vi "NO_NO_HumanDriveButtonReefCoralPositions.vi"() -> ()   [LabVIEW 2023]
uses:
  <vilib>/Rock Robotics/WPI/ThirdParty/JAS_Junk/TrajLib/Trajectory_Library.lvlib
  HumanGlobal.vi
panel:
  in  "DriverBoxRight":bool
  in  "DriverBoxLeft":bool
  in  "19-6 (bottom left)":bool
  in  "20-11 (top left)":bool
  in  "21-10 (outer)":bool
  in  "22-9 (top right)":bool
  in  "17-8 (bottom right)":bool
  in  "18-7 (inner)":bool
  out "DriveTraj":bool
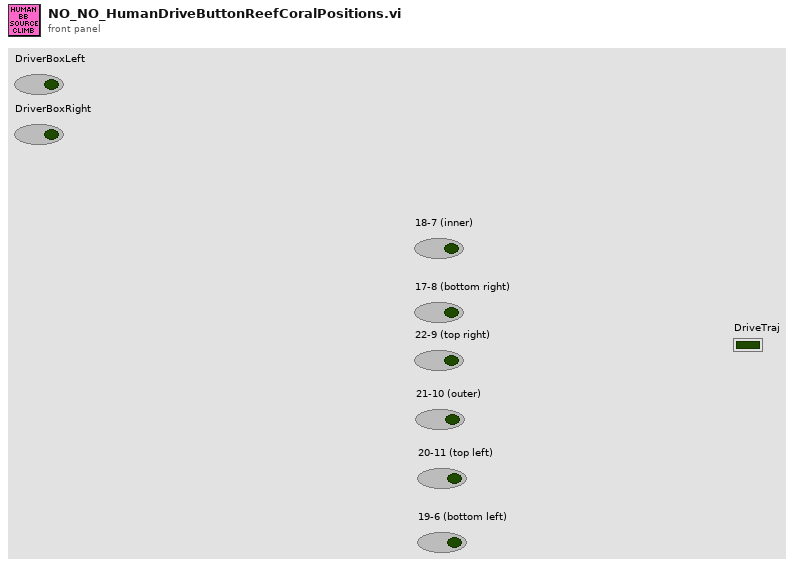
[diagram p1: front panel]
types:
  T1 = enum16{"No Trajectory", "18-7 (inner) left", "18-7 (inner) right", "17-8 (bottom right) left", "17-8 (bottom right) right", "22-9 (top right) left", "22-9 (top right) right", "21-10 (outer) left", "21-10 (outer) right", "20-11 (top left) left", "20-11 (top left) right", "19-6 (bottom left) left", "19-6 (bottom left) right"}
  T2 = typedef "WPI_DriverStationAllianceInfo.ctl" = enum16{"Red", "Blue", "Invalid"}
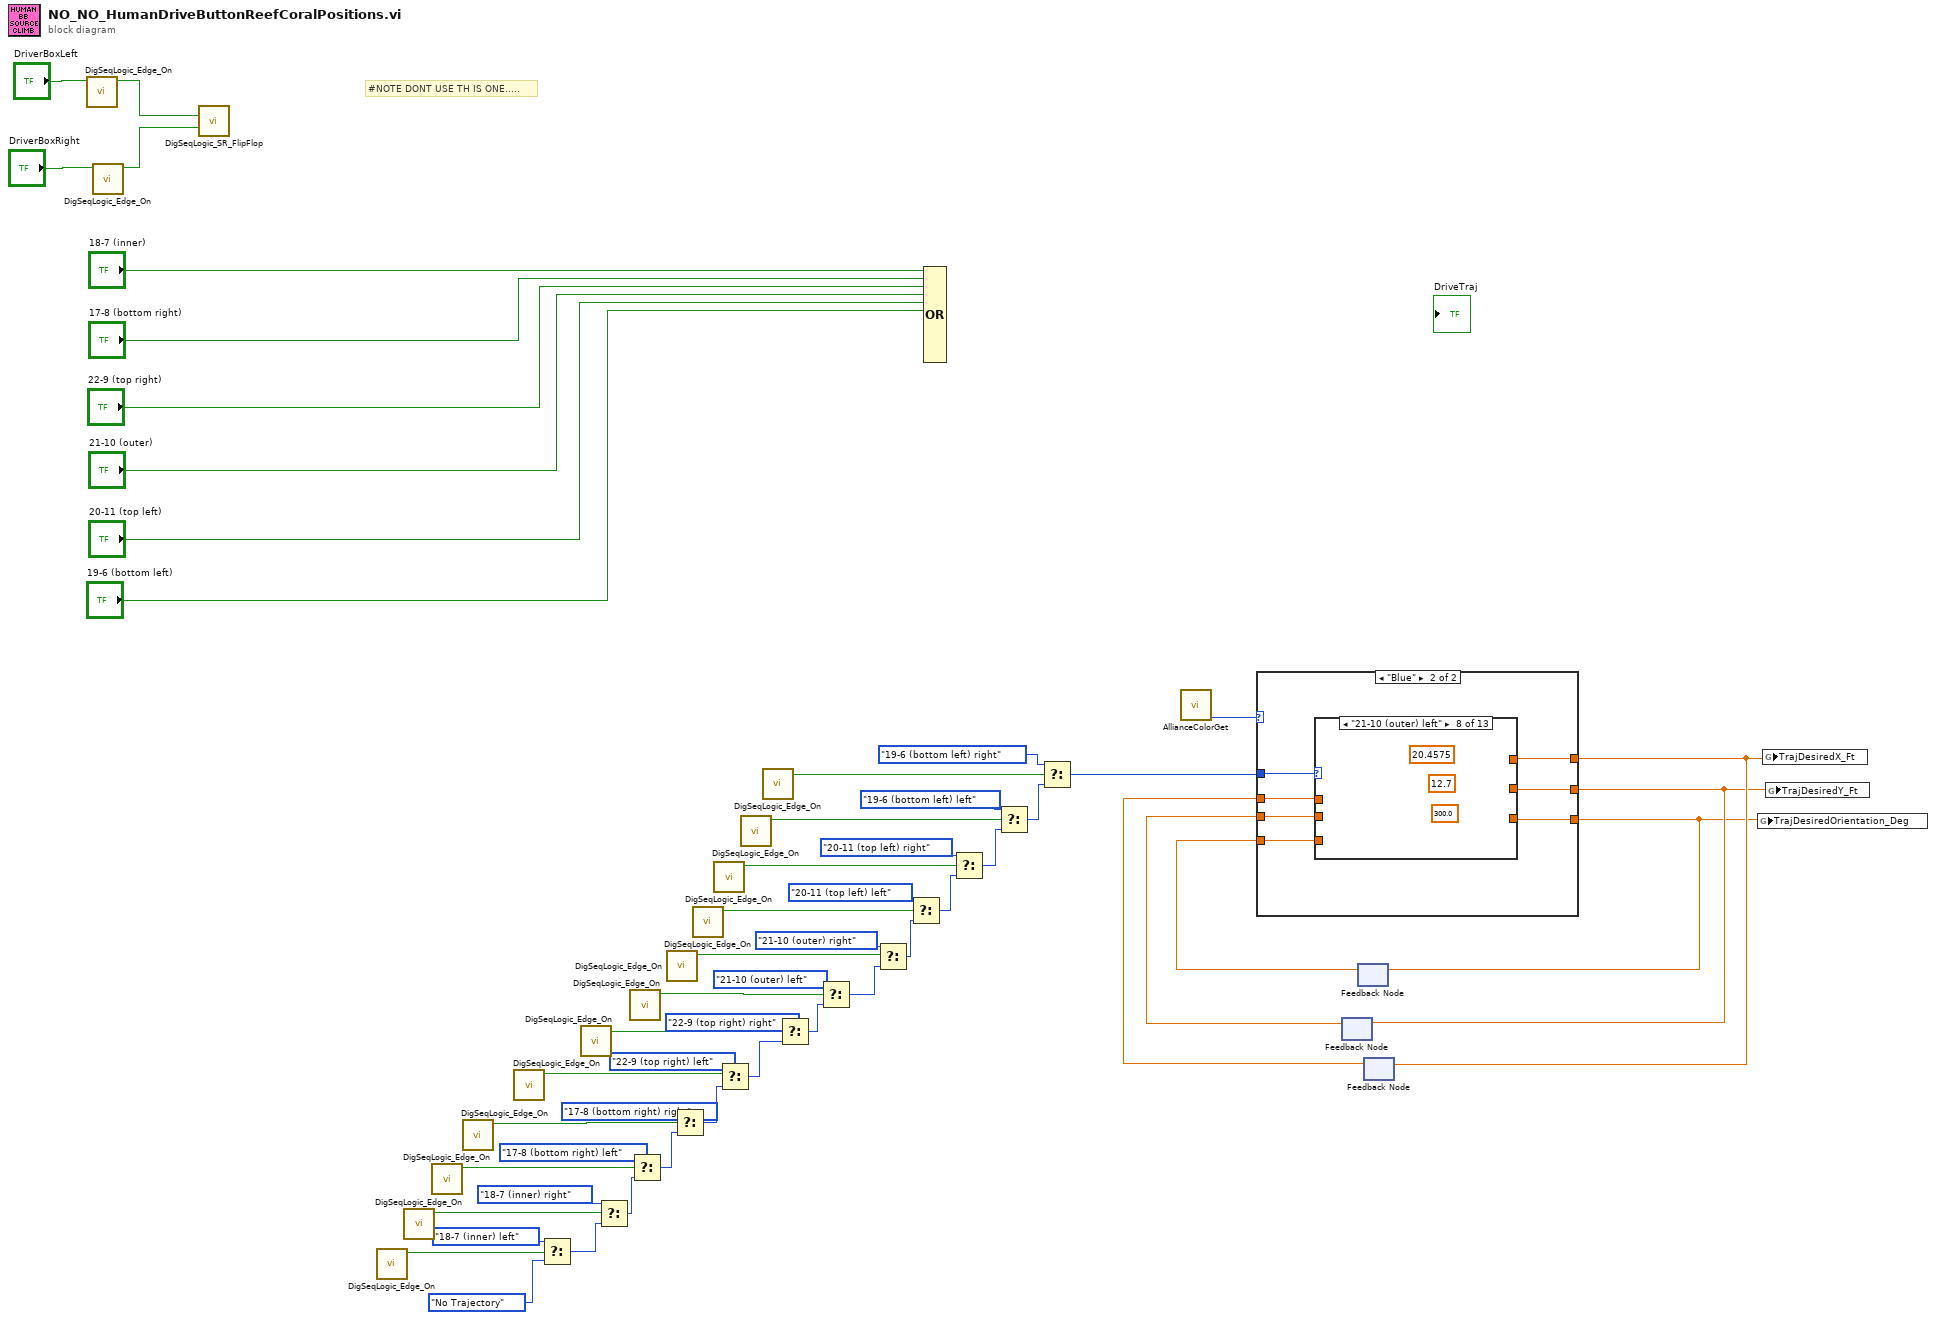
[diagram p0: block diagram]
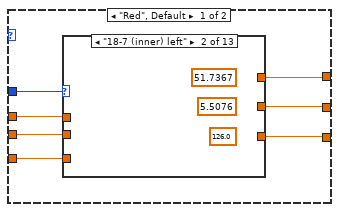
[diagram p2: hidden frame]
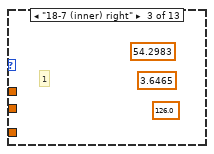
[diagram p4: hidden frame]
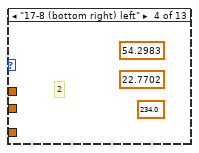
[diagram p5: hidden frame]
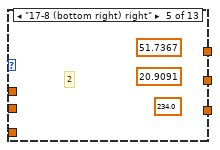
[diagram p6: hidden frame]
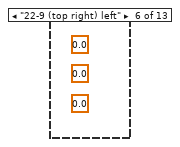
[diagram p7: hidden frame]
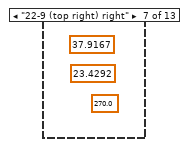
[diagram p8: hidden frame]
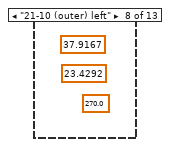
[diagram p9: hidden frame]
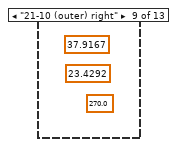
[diagram p10: hidden frame]
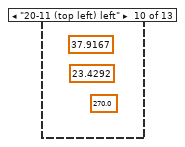
[diagram p11: hidden frame]
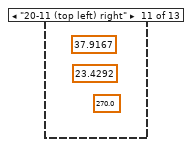
[diagram p12: hidden frame]
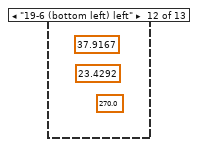
[diagram p13: hidden frame]
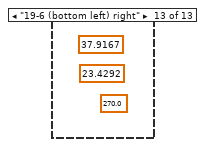
[diagram p14: hidden frame]
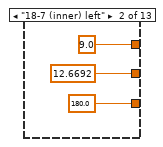
[diagram p16: hidden frame]
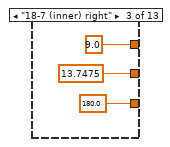
[diagram p17: hidden frame]
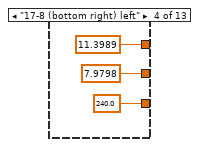
[diagram p18: hidden frame]
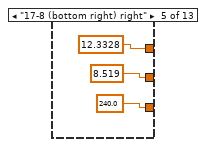
[diagram p19: hidden frame]
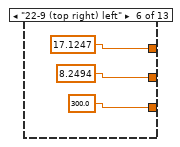
[diagram p20: hidden frame]
diagram:
  # "#NOTE DONT USE TH IS ONE....."
  n1 = call <vilib>:"DigSeqLogic_Edge_On.vi"("Input"="DriverBoxLeft") -> ("On Edge"=w27:bool)  [unwired: 10 in]
  n2 = call <vilib>:"DigSeqLogic_Edge_On.vi"("Input"="DriverBoxRight") -> ("On Edge"=w26:bool)  [unwired: 10 in]
  n3 = call <vilib>:"DigSeqLogic_SR_FlipFlop.vi"("Set"=w27, "Reset"=w26) -> ()  [unwired: 12 in, 2 out]
  n4 = call <vilib>:"DigSeqLogic_Edge_On.vi"() -> ("On Edge"=w25:bool)  [unwired: 11 in]
  n5 = call <vilib>:"DigSeqLogic_Edge_On.vi"() -> ("On Edge"=w19:bool)  [unwired: 11 in]
  n6 = call <vilib>:"DigSeqLogic_Edge_On.vi"() -> ("On Edge"=w18:bool)  [unwired: 11 in]
  n7 = call <vilib>:"DigSeqLogic_Edge_On.vi"() -> ("On Edge"=w17:bool)  [unwired: 11 in]
  n8 = call <vilib>:"DigSeqLogic_Edge_On.vi"() -> ("On Edge"=w16:bool)  [unwired: 11 in]
  n9 = Select(t=T1."18-7 (inner) left", s=w25, f=T1."No Trajectory") -> (s? t:f=w24:T1)
  n10 = call <vilib>:"DigSeqLogic_Edge_On.vi"() -> ("On Edge"=w15:bool)  [unwired: 11 in]
  n11 = Select(t=T1."18-7 (inner) right", s=w19, f=w24) -> (s? t:f=w23:T1)
  n12 = call <vilib>:"DigSeqLogic_Edge_On.vi"() -> ("On Edge"=w54:bool)  [unwired: 11 in]
  n13 = Select(t=T1."17-8 (bottom right) left", s=w18, f=w23) -> (s? t:f=w22:T1)
  n14 = call <vilib>:"DigSeqLogic_Edge_On.vi"() -> ("On Edge"=w48:bool)  [unwired: 11 in]
  n15 = Select(t=T1."17-8 (bottom right) right", s=w17, f=w22) -> (s? t:f=w21:T1)
  n16 = call <vilib>:"DigSeqLogic_Edge_On.vi"() -> ("On Edge"=w47:bool)  [unwired: 11 in]
  n17 = call <vilib>:"DigSeqLogic_Edge_On.vi"() -> ("On Edge"=w46:bool)  [unwired: 11 in]
  n18 = Select(t=T1."22-9 (top right) left", s=w16, f=w21) -> (s? t:f=w20:T1)
  n19 = call <vilib>:"DigSeqLogic_Edge_On.vi"() -> ("On Edge"=w45:bool)  [unwired: 11 in]
  n20 = call <vilib>:"DigSeqLogic_Edge_On.vi"() -> ("On Edge"=w44:bool)  [unwired: 11 in]
  n21 = Select(t=T1."22-9 (top right) right", s=w15, f=w20) -> (s? t:f=w14:T1)
  n22 = Select(t=T1."21-10 (outer) left", s=w54, f=w14) -> (s? t:f=w53:T1)
  n23 = Select(t=T1."21-10 (outer) right", s=w48, f=w53) -> (s? t:f=w52:T1)
  n24 = Select(t=T1."20-11 (top left) left", s=w47, f=w52) -> (s? t:f=w51:T1)
  n25 = Compound Arithmetic op=OR("18-7 (inner)", "17-8 (bottom right)", "22-9 (top right)", "21-10 (outer)", "20-11 (top left)", "19-6 (bottom left)") -> ()  [unwired: 6 in, 1 out]
  n26 = Select(t=T1."20-11 (top left) right", s=w46, f=w51) -> (s? t:f=w50:T1)
  n27 = Select(t=T1."19-6 (bottom left) left", s=w45, f=w50) -> (s? t:f=w49:T1)
  n28 = Select(t=T1."19-6 (bottom left) right", s=w44, f=w49) -> (s? t:f=w43:T1)
  n29 = call "AllianceColorGet.vi"() -> ("AllianceColor"=w36:T2)  [unwired: 11 in]
  n30 = feedback #1() -> (w39:dbl)  [unwired: 1 in]
  n31 = feedback #2() -> (w37:dbl)  [unwired: 1 in]
  n32 = feedback #3() -> (w41:dbl)  [unwired: 1 in]
  n33 = case shown="\"Blue\"" w36 {
    tunnel: w43 -> [w61 w71]
    tunnel: [w60 w70] -> w42
    tunnel: w41 -> [w55 w69]
    tunnel: [w59 w68] -> w40
    tunnel: w39 -> [w56 w67]
    tunnel: [w58 w66] -> w38
    tunnel: w37 -> [w57 w65]
    frame "Red", Default {
      n34 = case shown="\"18-7 (inner) left\"" w61 {
        tunnel: [w64 _ _ _ _ _ _ _ _ _ _ _ _] -> w60
        tunnel: [w63 _ _ _ _ _ _ _ _ _ _ _ _] -> w59
        tunnel: [w62 _ _ _ _ _ _ _ _ _ _ _ _] -> w58
        tunnel: w55 -> [w64 _ _ _ _ _ _ _ _ _ _ _ _]
        tunnel: w56 -> [w63 _ _ _ _ _ _ _ _ _ _ _ _]
        tunnel: w57 -> [w62 _ _ _ _ _ _ _ _ _ _ _ _]
        frame "No Trajectory" {
        }
        frame "18-7 (inner) left" {
          (unwired) 126.0 ("TrajDesiredOrientation_Deg")
          (unwired) 5.5076 ("TrajDesiredY_Ft")
          (unwired) 51.7367 ("TrajDesiredX_Ft")
        }
        frame "18-7 (inner) right" {
          (unwired) 126.0 ("TrajDesiredOrientation_Deg")
          (unwired) 3.6465 ("TrajDesiredY_Ft")
          (unwired) 54.2983 ("TrajDesiredX_Ft")
          # "1"
        }
        frame "17-8 (bottom right) left" {
          (unwired) 234.0 ("TrajDesiredOrientation_Deg")
          (unwired) 22.7702 ("TrajDesiredY_Ft")
          (unwired) 54.2983 ("TrajDesiredX_Ft")
          # "2"
        }
        frame "17-8 (bottom right) right" {
          (unwired) 234.0 ("TrajDesiredOrientation_Deg")
          (unwired) 20.9091 ("TrajDesiredY_Ft")
          (unwired) 51.7367 ("TrajDesiredX_Ft")
          # "2"
        }
        frame "22-9 (top right) left" {
          (unwired) 0.0 ("TrajDesiredOrientation_Deg")
          (unwired) 0.0 ("TrajDesiredY_Ft")
          (unwired) 0.0 ("TrajDesiredX_Ft")
        }
        frame "22-9 (top right) right" {
          (unwired) 270.0 ("TrajDesiredOrientation_Deg")
          (unwired) 23.4292 ("TrajDesiredY_Ft")
          (unwired) 37.9167 ("TrajDesiredX_Ft")
        }
        frame "21-10 (outer) left" {
          (unwired) 270.0 ("TrajDesiredOrientation_Deg")
          (unwired) 23.4292 ("TrajDesiredY_Ft")
          (unwired) 37.9167 ("TrajDesiredX_Ft")
        }
        frame "21-10 (outer) right" {
          (unwired) 270.0 ("TrajDesiredOrientation_Deg")
          (unwired) 23.4292 ("TrajDesiredY_Ft")
          (unwired) 37.9167 ("TrajDesiredX_Ft")
        }
        frame "20-11 (top left) left" {
          (unwired) 270.0 ("TrajDesiredOrientation_Deg")
          (unwired) 23.4292 ("TrajDesiredY_Ft")
          (unwired) 37.9167 ("TrajDesiredX_Ft")
        }
        frame "20-11 (top left) right" {
          (unwired) 270.0 ("TrajDesiredOrientation_Deg")
          (unwired) 23.4292 ("TrajDesiredY_Ft")
          (unwired) 37.9167 ("TrajDesiredX_Ft")
        }
        frame "19-6 (bottom left) left" {
          (unwired) 270.0 ("TrajDesiredOrientation_Deg")
          (unwired) 23.4292 ("TrajDesiredY_Ft")
          (unwired) 37.9167 ("TrajDesiredX_Ft")
        }
        frame "19-6 (bottom left) right" {
          (unwired) 270.0 ("TrajDesiredOrientation_Deg")
          (unwired) 23.4292 ("TrajDesiredY_Ft")
          (unwired) 37.9167 ("TrajDesiredX_Ft")
        }
      }
    }
    frame "Blue" {
      n35 = case shown="\"21-10 (outer) left\"" w71 {
        tunnel: [w74 9.0 ("TrajDesiredX_Ft") 9.0 ("TrajDesiredX_Ft") 11.3989 ("TrajDesiredX_Ft") 12.3328 ("TrajDesiredX_Ft") 17.1247 ("TrajDesiredX_Ft") 18.0586 ("TrajDesiredX_Ft") _ _ _ _ _ _] -> w70
        tunnel: [w73 12.6692 ("TrajDesiredY_Ft") 13.7475 ("TrajDesiredY_Ft") 7.9798 ("TrajDesiredY_Ft") 8.519 ("TrajDesiredY_Ft") 8.2494 ("TrajDesiredY_Ft") 8.51 ("TrajDesiredY_Ft") _ _ _ _ _ _] -> w68
        tunnel: [w72 180.0 ("TrajDesiredOrientation_Deg") 180.0 ("TrajDesiredOrientation_Deg") 240.0 ("TrajDesiredOrientation_Deg") 240.0 ("TrajDesiredOrientation_Deg") 300.0 ("TrajDesiredOrientation_Deg") 300.0 ("TrajDesiredOrientation_Deg") _ _ _ _ _ _] -> w66
        tunnel: w69 -> [w74 _ _ _ _ _ _ _ _ _ _ _ _]
        tunnel: w67 -> [w73 _ _ _ _ _ _ _ _ _ _ _ _]
        tunnel: w65 -> [w72 _ _ _ _ _ _ _ _ _ _ _ _]
        frame "No Trajectory" {
        }
        frame "18-7 (inner) left" {
        }
        frame "18-7 (inner) right" {
        }
        frame "17-8 (bottom right) left" {
        }
        frame "17-8 (bottom right) right" {
        }
        frame "22-9 (top right) left" {
        }
        frame "22-9 (top right) right" {
        }
        frame "21-10 (outer) left" {
          (unwired) 300.0 ("TrajDesiredOrientation_Deg")
          (unwired) 12.7 ("TrajDesiredY_Ft")
          (unwired) 20.4575 ("TrajDesiredX_Ft")
        }
        frame "21-10 (outer) right" {
          (unwired) 300.0 ("TrajDesiredOrientation_Deg")
          (unwired) 8.51 ("TrajDesiredY_Ft")
          (unwired) 18.0586 ("TrajDesiredX_Ft")
        }
        frame "20-11 (top left) left" {
          (unwired) 300.0 ("TrajDesiredOrientation_Deg")
          (unwired) 8.51 ("TrajDesiredY_Ft")
          (unwired) 18.0586 ("TrajDesiredX_Ft")
        }
        frame "20-11 (top left) right" {
          (unwired) 300.0 ("TrajDesiredOrientation_Deg")
          (unwired) 8.51 ("TrajDesiredY_Ft")
          (unwired) 18.0586 ("TrajDesiredX_Ft")
        }
        frame "19-6 (bottom left) left" {
          (unwired) 300.0 ("TrajDesiredOrientation_Deg")
          (unwired) 8.51 ("TrajDesiredY_Ft")
          (unwired) 18.0586 ("TrajDesiredX_Ft")
        }
        frame "19-6 (bottom left) right" {
          (unwired) 300.0 ("TrajDesiredOrientation_Deg")
          (unwired) 8.51 ("TrajDesiredY_Ft")
          (unwired) 18.0586 ("TrajDesiredX_Ft")
        }
      }
    }
  }
  n36 = feedback-in #1(w40) -> ()
  n37 = feedback-in #2(w38) -> ()
  n38 = feedback-in #3(w42) -> ()
  n39 = global write "HumanGlobal.vi" "TrajDesiredOrientation_Deg"(w38) -> ()
  n40 = global write "HumanGlobal.vi" "TrajDesiredX_Ft"(w42) -> ()
  n41 = global write "HumanGlobal.vi" "TrajDesiredY_Ft"(w40) -> ()
